vi "Benchmark SV Send  LV2012 - NI Verified - 1000 Byte - 1Var - 10num.vi"() -> ()   [LabVIEW 2015]
uses:
  <vilib>/Platform/TimedLoop/XDataNode/timing_clust.ctl
  <vilib>/Platform/TimedLoop/XDataNode/nitl_modes.ctl
  <vilib>/Platform/TimedLoop/XDataNode/wakeup.ctl
  <vilib>/platform/TimedLoop/XDataNode/XDataNode.xnode
  <vilib>/Platform/TimedLoop/XDataNode/XDNodeRunTimeDep.lvlib
panel:
  out "Time":u32
  out "Tries":u32
  out "Average Delay (ms)":dbl
  out "Delay (ms)":u32
  in  "stop":bool
  # "Overview:  Coding that exemplifies how to benchmark the communication of Shared Variables.\nRequirements: LabVIEW 2012 or compatible\nInstructions:\n1.  Run the \"Benchmark SV Receive LV2012 - NI Verified.vi\"\n2. Run this VI\n3. Watch the amount of time it takes to communicate\n4. Stop both VIs"
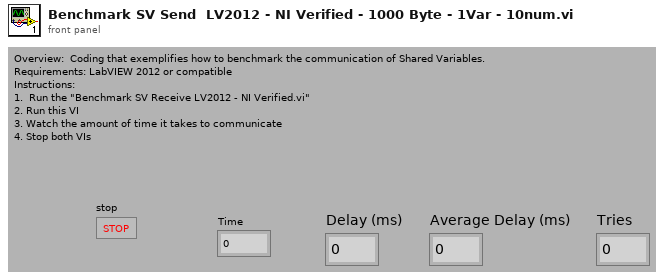
[diagram p1: front panel]
types:
  T1 = typedef "XDNodeRunTimeDep.lvlib/timing_clust.ctl" = cluster{"Expected End [f-1]":u64, "Actual End [f-1]":u64, "Finished Late? [f-1]":bool, "Expected End [i-1]":u64, "Actual End [i-1]":u64, "Finished Late? [i-1]":bool, "Expected Start [i]":u64, "Actual Start [i]":u64, "Expected Start [f]":u64, "Actual Start [f]":u64, "Source Name":string, "Structure Name":string, "Period":i64, "Deadline":i64, "Offset":i64, "Start":i64, "Priority":i32, "Timeout":i32, "Mode":T2, "Wakeup Reason":T3, "Error":errorcluster, "Source Type":string, "Secondary Source Type":string, "Global End Time":u64, "Global Start Time":u64, "Frame Duration":u64, "Iteration Duration":u64, "Assigned CPU":i32, "I/O Scan Engine Mode":u32}
  T2 = typedef "XDNodeRunTimeDep.lvlib/nitl_modes.ctl" = enum32{"No Change", "Process missed periods, maintain original phase", "Discard missed periods, maintain original phase", "Process missed periods, ignore original phase", "Discard missed periods, ignore original phase"}
  T3 = typedef "XDNodeRunTimeDep.lvlib/wakeup.ctl" = enum32{"Normal", "Aborted", "Asynchronous wakeup", "Timing source error", "Timed loop error", "Timeout"}
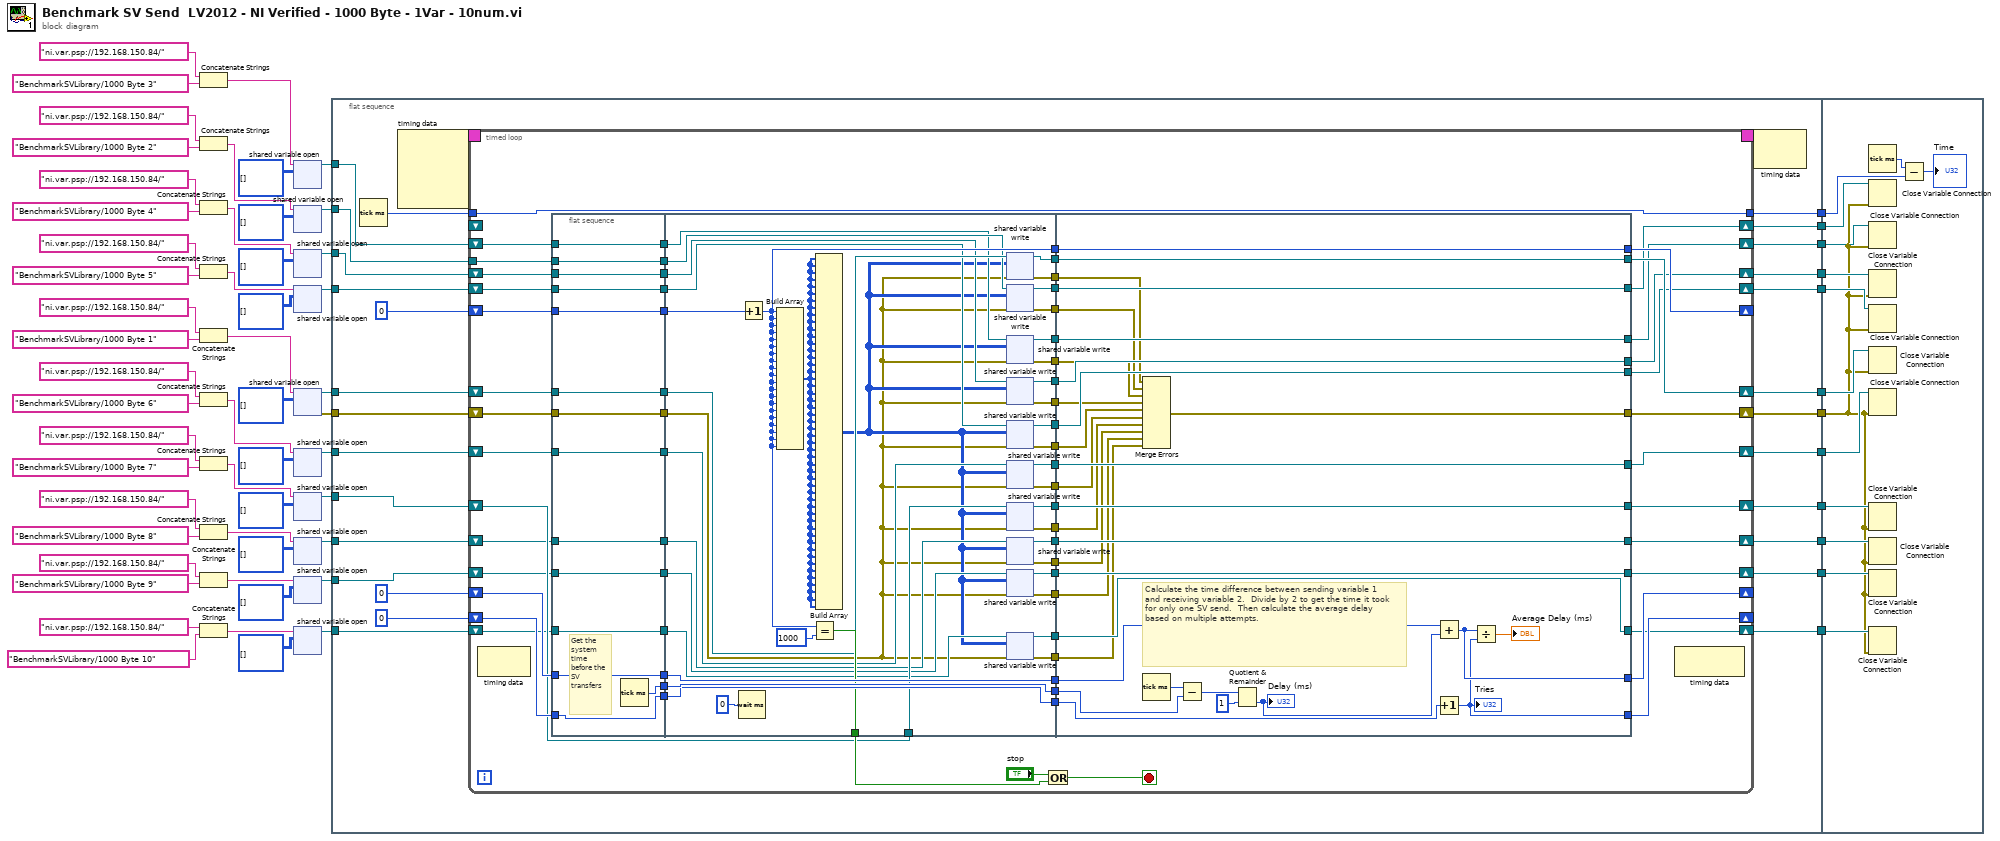
[diagram p0: block diagram]
diagram:
  n1 = Concatenate Strings("ni.var.psp://192.168.150.84/" ("string"), "BenchmarkSVLibrary/1000 Byte 3") -> (w47:string)
  n2 = Concatenate Strings("ni.var.psp://192.168.150.84/" ("string"), "BenchmarkSVLibrary/1000 Byte 2") -> (w54:string)
  n3 = Concatenate Strings("ni.var.psp://192.168.150.84/" ("string"), "BenchmarkSVLibrary/1000 Byte 4") -> (w46:string)
  n4 = Concatenate Strings("ni.var.psp://192.168.150.84/" ("string"), "BenchmarkSVLibrary/1000 Byte 5") -> (w40:string)
  n5 = Concatenate Strings("ni.var.psp://192.168.150.84/" ("string"), "BenchmarkSVLibrary/1000 Byte 1") -> (w60:string)
  n6 = Concatenate Strings("ni.var.psp://192.168.150.84/" ("string"), "BenchmarkSVLibrary/1000 Byte 6") -> (w39:string)
  n7 = Concatenate Strings("ni.var.psp://192.168.150.84/" ("string"), "BenchmarkSVLibrary/1000 Byte 7") -> (w34:string)
  n8 = Concatenate Strings("ni.var.psp://192.168.150.84/" ("string"), "BenchmarkSVLibrary/1000 Byte 8") -> (w33:string)
  n9 = Concatenate Strings("ni.var.psp://192.168.150.84/" ("string"), "BenchmarkSVLibrary/1000 Byte 9") -> (w28:string)
  n10 = Concatenate Strings("ni.var.psp://192.168.150.84/" ("string"), "BenchmarkSVLibrary/1000 Byte 10") -> (w27:string)
  n11 = shared-variable-open(w47, i32[][] [] ("appended array")) -> (w23:refnum<k21>)  [unwired: 2 in, 1 out]
  n12 = shared-variable-open(w54, i32[][] [] ("appended array")) -> (w24:refnum<k21>)  [unwired: 2 in, 1 out]
  n13 = shared-variable-open(w46, i32[][] [] ("appended array")) -> (w22:refnum<k21>)  [unwired: 2 in, 1 out]
  n14 = shared-variable-open(w40, i32[][] [] ("appended array")) -> (w21:refnum<k21>)  [unwired: 2 in, 1 out]
  n15 = shared-variable-open(w60, i32[][] [] ("appended array")) -> (w56:refnum<k21>, w57:errorcluster)  [unwired: 2 in]
  n16 = shared-variable-open(w39, i32[][] [] ("appended array")) -> (w20:refnum<k21>)  [unwired: 2 in, 1 out]
  n17 = shared-variable-open(w34, i32[][] [] ("appended array")) -> (w19:refnum<k21>)  [unwired: 2 in, 1 out]
  n18 = shared-variable-open(w33, i32[][] [] ("appended array")) -> (w18:refnum<k21>)  [unwired: 2 in, 1 out]
  n19 = shared-variable-open(w28, i32[][] [] ("appended array")) -> (w17:refnum<k21>)  [unwired: 2 in, 1 out]
  n20 = shared-variable-open(w27, i32[][] [] ("appended array")) -> (w16:refnum<k21>)  [unwired: 2 in, 1 out]
  n21 = flat-sequence {
    tunnel: [w89] -> w59
    tunnel: [w88] -> w58
    tunnel: w57 -> [w87]
    tunnel: w56 -> [w86]
    tunnel: [w85] -> w55
    tunnel: w24 -> [w81]
    tunnel: w23 -> [w80]
    tunnel: w22 -> [w79]
    tunnel: w21 -> [w78]
    tunnel: w20 -> [w77]
    tunnel: w19 -> [w76]
    tunnel: w18 -> [w75]
    tunnel: w17 -> [w74]
    tunnel: w16 -> [w73]
    tunnel: [w72] -> w9
    tunnel: [w71] -> w8
    tunnel: [w70] -> w7
    tunnel: [w69] -> w6
    tunnel: [w68] -> w5
    tunnel: [w67] -> w4
    tunnel: [w66] -> w3
    tunnel: [w65] -> w2
    tunnel: [w64] -> w1
    tunnel: w59 -> [w254]
    tunnel: w58 -> [w267]
    tunnel: w55 -> [w264]
    tunnel: w9 -> [w263]
    tunnel: w8 -> [w262]
    tunnel: w7 -> [w261]
    tunnel: w6 -> [w260]
    tunnel: w5 -> [w259]
    tunnel: w4 -> [w258]
    tunnel: w3 -> [w257]
    tunnel: w2 -> [w256]
    tunnel: w1 -> [w255]
    frame #0 {
      n22 = Tick Count (ms)() -> (millisecond timer value=w84:u32)
      n23 = node-c288() -> (w83:T1)  [unwired: 4 in]
      n24 = timed-loop {
        shift-right: [w162] -> _
        shift-left: u32 0 -> [w156]
        shift-right: [w161] -> _
        shift-left: u32 0 -> [w157]
        shift-right: [w153] -> _
        shift-left: 0 -> [w154]
        shift-right: [w145] -> w89
        shift-left: w87 -> [w140]
        shift-right: [w144] -> w88
        shift-left: w86 -> [w141]
        tunnel: [w139] -> w85
        tunnel: w84 -> [w139]
        timing: w83 -> [_]
        timing-out: [_] -> w82
        tunnel: w81 -> [w137]
        shift-right: [w136] -> w72
        shift-left: _ -> [_]
        shift-right: [w132] -> w71
        shift-left: w80 -> [w133]
        shift-right: [w128] -> w70
        shift-left: w79 -> [w129]
        shift-right: [w124] -> w69
        shift-left: w78 -> [w125]
        shift-right: [w120] -> w68
        shift-left: w77 -> [w121]
        shift-right: [w117] -> w67
        shift-left: w76 -> [w118]
        shift-right: [w113] -> w66
        shift-left: w75 -> [w114]
        shift-right: [w109] -> w65
        shift-left: w74 -> [w111]
        shift-right: [w105] -> w64
        shift-left: w73 -> [w106]
        stop <- w152 stop-if-true
        n25 = node-c288() -> ()  [unwired: 1 in, 1 out]
        n26 = flat-sequence {
          tunnel: [w176] -> w160
          tunnel: [w178] -> w159
          tunnel: [w177] -> w158
          tunnel: [w175] -> w155
          tunnel: w156 -> [w178]
          tunnel: w157 -> [w177]
          tunnel: w154 -> [w175]
          tunnel: [w174] -> w142
          tunnel: w141 -> [w174]
          tunnel: w140 -> [w165]
          tunnel: [w173] -> w138
          tunnel: w137 -> [w173]
          tunnel: [w172] -> w134
          tunnel: w133 -> [w172]
          tunnel: [w171] -> w130
          tunnel: w129 -> [w171]
          tunnel: [w170] -> w126
          tunnel: w125 -> [w170]
          tunnel: [w169] -> w122
          tunnel: w121 -> [w169]
          tunnel: [w168] -> w115
          tunnel: w114 -> [w168]
          tunnel: w111 -> [w167]
          tunnel: [w167] -> w110
          tunnel: [w166] -> w107
          tunnel: w106 -> [w166]
          tunnel: [w165] -> w103
          tunnel: [w219] -> w149
          tunnel: [w218] -> w148
          tunnel: [w217] -> w147
          tunnel: w160 -> [w219]
          tunnel: w159 -> [w218]
          tunnel: w158 -> [w217]
          tunnel: w155 -> [w216]
          tunnel: [w213] -> w146
          tunnel: [w212] -> w150
          tunnel: [w211] -> w143
          tunnel: w142 -> [w210]
          tunnel: w138 -> [w208]
          tunnel: [w207] -> w135
          tunnel: w134 -> [w206]
          tunnel: [w205] -> w131
          tunnel: w130 -> [w204]
          tunnel: [w203] -> w127
          tunnel: w126 -> [w202]
          tunnel: [w201] -> w123
          tunnel: w122 -> [w200]
          tunnel: [w199] -> w119
          tunnel: w118 -> [w198]
          tunnel: [w197] -> w116
          tunnel: w115 -> [w196]
          tunnel: [w195] -> w112
          tunnel: w110 -> [w194]
          tunnel: [w193] -> w108
          tunnel: w107 -> [w192]
          tunnel: [w191] -> w104
          tunnel: w103 -> [w189]
          tunnel: [w188] -> w102
          tunnel: [w187] -> w101
          tunnel: [w186] -> w100
          tunnel: [w185] -> w99
          tunnel: [w184] -> w98
          tunnel: [w183] -> w97
          tunnel: [w182] -> w96
          tunnel: [w181] -> w95
          tunnel: [w180] -> w94
          tunnel: [w179] -> w93
          tunnel: w149 -> [w250]
          tunnel: [w243] -> w162
          tunnel: w148 -> [w245]
          tunnel: [w242] -> w161
          tunnel: w147 -> [w249]
          tunnel: w146 -> [w241]
          tunnel: [w241] -> w153
          tunnel: [w220] -> w145
          tunnel: [w240] -> w144
          tunnel: w143 -> [w240]
          tunnel: [w239] -> w136
          tunnel: w135 -> [w239]
          tunnel: [w238] -> w132
          tunnel: w131 -> [w238]
          tunnel: [w237] -> w128
          tunnel: w127 -> [w237]
          tunnel: [w236] -> w124
          tunnel: w123 -> [w236]
          tunnel: [w235] -> w120
          tunnel: w119 -> [w235]
          tunnel: [w234] -> w117
          tunnel: w116 -> [w234]
          tunnel: [w233] -> w113
          tunnel: w112 -> [w233]
          tunnel: [w232] -> w109
          tunnel: w108 -> [w232]
          tunnel: [w231] -> w105
          tunnel: w104 -> [w231]
          tunnel: w102 -> [w230]
          tunnel: w101 -> [w229]
          tunnel: w100 -> [w228]
          tunnel: w99 -> [w227]
          tunnel: w98 -> [w226]
          tunnel: w97 -> [w225]
          tunnel: w96 -> [w224]
          tunnel: w95 -> [w223]
          tunnel: w94 -> [w222]
          tunnel: w93 -> [w221]
          frame #0 {
            # "Get the system time before the SV transfers"
            n27 = Tick Count (ms)() -> (millisecond timer value=w176:u32)
          }
          frame #1 {
            n28 = Wait (ms)(milliseconds to wait=u32 0) -> ()  [unwired: 1 out]
            n29 = Increment(x=w216) -> (x+1=w213:i32)
            n30 = Build Array(w213, w213, w213, w213, w213, w213, w213, w213, w213, w213, w213, w213, w213, w213, w213, w213, w213, w213, w213, w213) -> (w214:i32[])
            n31 = Equal?(x=w213, y=1000) -> (x = y?=w212:bool)
            n32 = Build Array(w214, w214, w214, w214, w214, w214, w214, w214, w214, w214, w214, w214, w214, w214, w214, w214, w214, w214, w214, w214, w214, w214, w214, w214, w214, w214, w214, w214, w214, w214, w214, w214, w214, w214, w214, w214, w214, w214, w214, w214, w214, w214, w214, w214, w214, w214, w214, w214, w214, w214) -> (w190:i32[][])
            n33 = shared-variable-write(w210, w189, w190) -> (w211:refnum<k21>, w188:errorcluster)
            n34 = shared-variable-write(w208, w189, w190) -> (w207:refnum<k21>, w187:errorcluster)
            n35 = shared-variable-write(w206, w189, w190) -> (w205:refnum<k21>, w186:errorcluster)
            n36 = shared-variable-write(w204, w189, w190) -> (w203:refnum<k21>, w185:errorcluster)
            n37 = shared-variable-write(w202, w189, w190) -> (w201:refnum<k21>, w184:errorcluster)
            n38 = shared-variable-write(w200, w189, w190) -> (w199:refnum<k21>, w183:errorcluster)
            n39 = shared-variable-write(w198, w189, w190) -> (w197:refnum<k21>, w182:errorcluster)
            n40 = shared-variable-write(w196, w189, w190) -> (w195:refnum<k21>, w181:errorcluster)
            n41 = shared-variable-write(w194, w189, w190) -> (w193:refnum<k21>, w180:errorcluster)
            n42 = shared-variable-write(w192, w189, w190) -> (w191:refnum<k21>, w179:errorcluster)
          }
          frame #2 {
            # "Calculate the time difference between sending variable 1 and receiving variable 2.  Divide by 2 to get the time it took for only one SV send.  Then calculate the average delay based on multiple attempts."
            n43 = Merge Errors(w230, w229, w228, w227, w226, w225, w224, w223, w222, w221) -> (w220:errorcluster)
            n44 = Tick Count (ms)() -> (millisecond timer value=w251:u32)
            n45 = Subtract(x=w251, y=w250) -> (x-y=w248:u32)
            n46 = Quotient & Remainder(x=w248, y=u32 1) -> (floor(x/y)=w246:u32)  [unwired: 1 out]
            "Delay (ms)" <- w246
            n47 = Add(x=w245, y=w246) -> (x+y=w243:u32)
            n48 = Increment(x=w249) -> (x+1=w242:u32)
            "Tries" <- w242
            n49 = Divide(x=w243, y=w242) -> (x/y=→"Average Delay (ms)":dbl)
          }
        }
        n50 = Or(x="stop", y=w150) -> (x .or. y?=w152:bool)
        n51 = node-c288() -> ()  [unwired: 1 in, 1 out]
      }
      n52 = node-c288(w82) -> ()  [unwired: 1 out]
    }
    frame #1 {
      n53 = Tick Count (ms)() -> (millisecond timer value=w266:u32)
      n54 = Close Variable Connection(8:w254, 11:w263) -> ()  [unwired: 1 out]
      n55 = Close Variable Connection(8:w254, 11:w262) -> ()  [unwired: 1 out]
      n56 = Close Variable Connection(8:w254, 11:w261) -> ()  [unwired: 1 out]
      n57 = Close Variable Connection(8:w254, 11:w260) -> ()  [unwired: 1 out]
      n58 = Close Variable Connection(8:w254, 11:w267) -> ()  [unwired: 1 out]
      n59 = Close Variable Connection(8:w254, 11:w259) -> ()  [unwired: 1 out]
      n60 = Close Variable Connection(8:w254, 11:w258) -> ()  [unwired: 1 out]
      n61 = Close Variable Connection(8:w254, 11:w257) -> ()  [unwired: 1 out]
      n62 = Close Variable Connection(8:w254, 11:w256) -> ()  [unwired: 1 out]
      n63 = Close Variable Connection(8:w254, 11:w255) -> ()  [unwired: 1 out]
      n64 = Subtract(x=w266, y=w264) -> (x-y=→"Time":u32)
    }
  }
